vi "VPA QC Pressure Test.vi"(7 "DAQ Q":T1, 9 "DAQ Ref Cluster":T2, 10 "State Cluster":T3) -> (2 "State Cluster Out":T3)   [LabVIEW 2013]
uses:
  Controls/VPA QC State Data Cluster.ctl
  Controls/VPA QC General Cluster.ctl
  Controls/VPA QC State Enum.ctl
  Controls/VPA QC Bool Cluster.ctl
  Controls/VPA QC DAQ Ref Cluster.ctl
  Controls/VPA QC DAQ Q.ctl
  Controls/VPA QC DAQ Cmd Enum.ctl
panel:
  in  "Cancel":bool
  in  "Save":bool
  in  "Stop Logging":bool
  in  "Log":bool
  out "Pressure Test":dbl[][](graph)
  # "Pressure Verification Test"
  # "1. In pressure control mode, ramp to 95% max pressure."
  # "2. Start logging"
  # "3. Crack the external valve enough to allow the cylinders to transition twice."
  # "Assembly Checklist"
  # "Assembly Checklist"
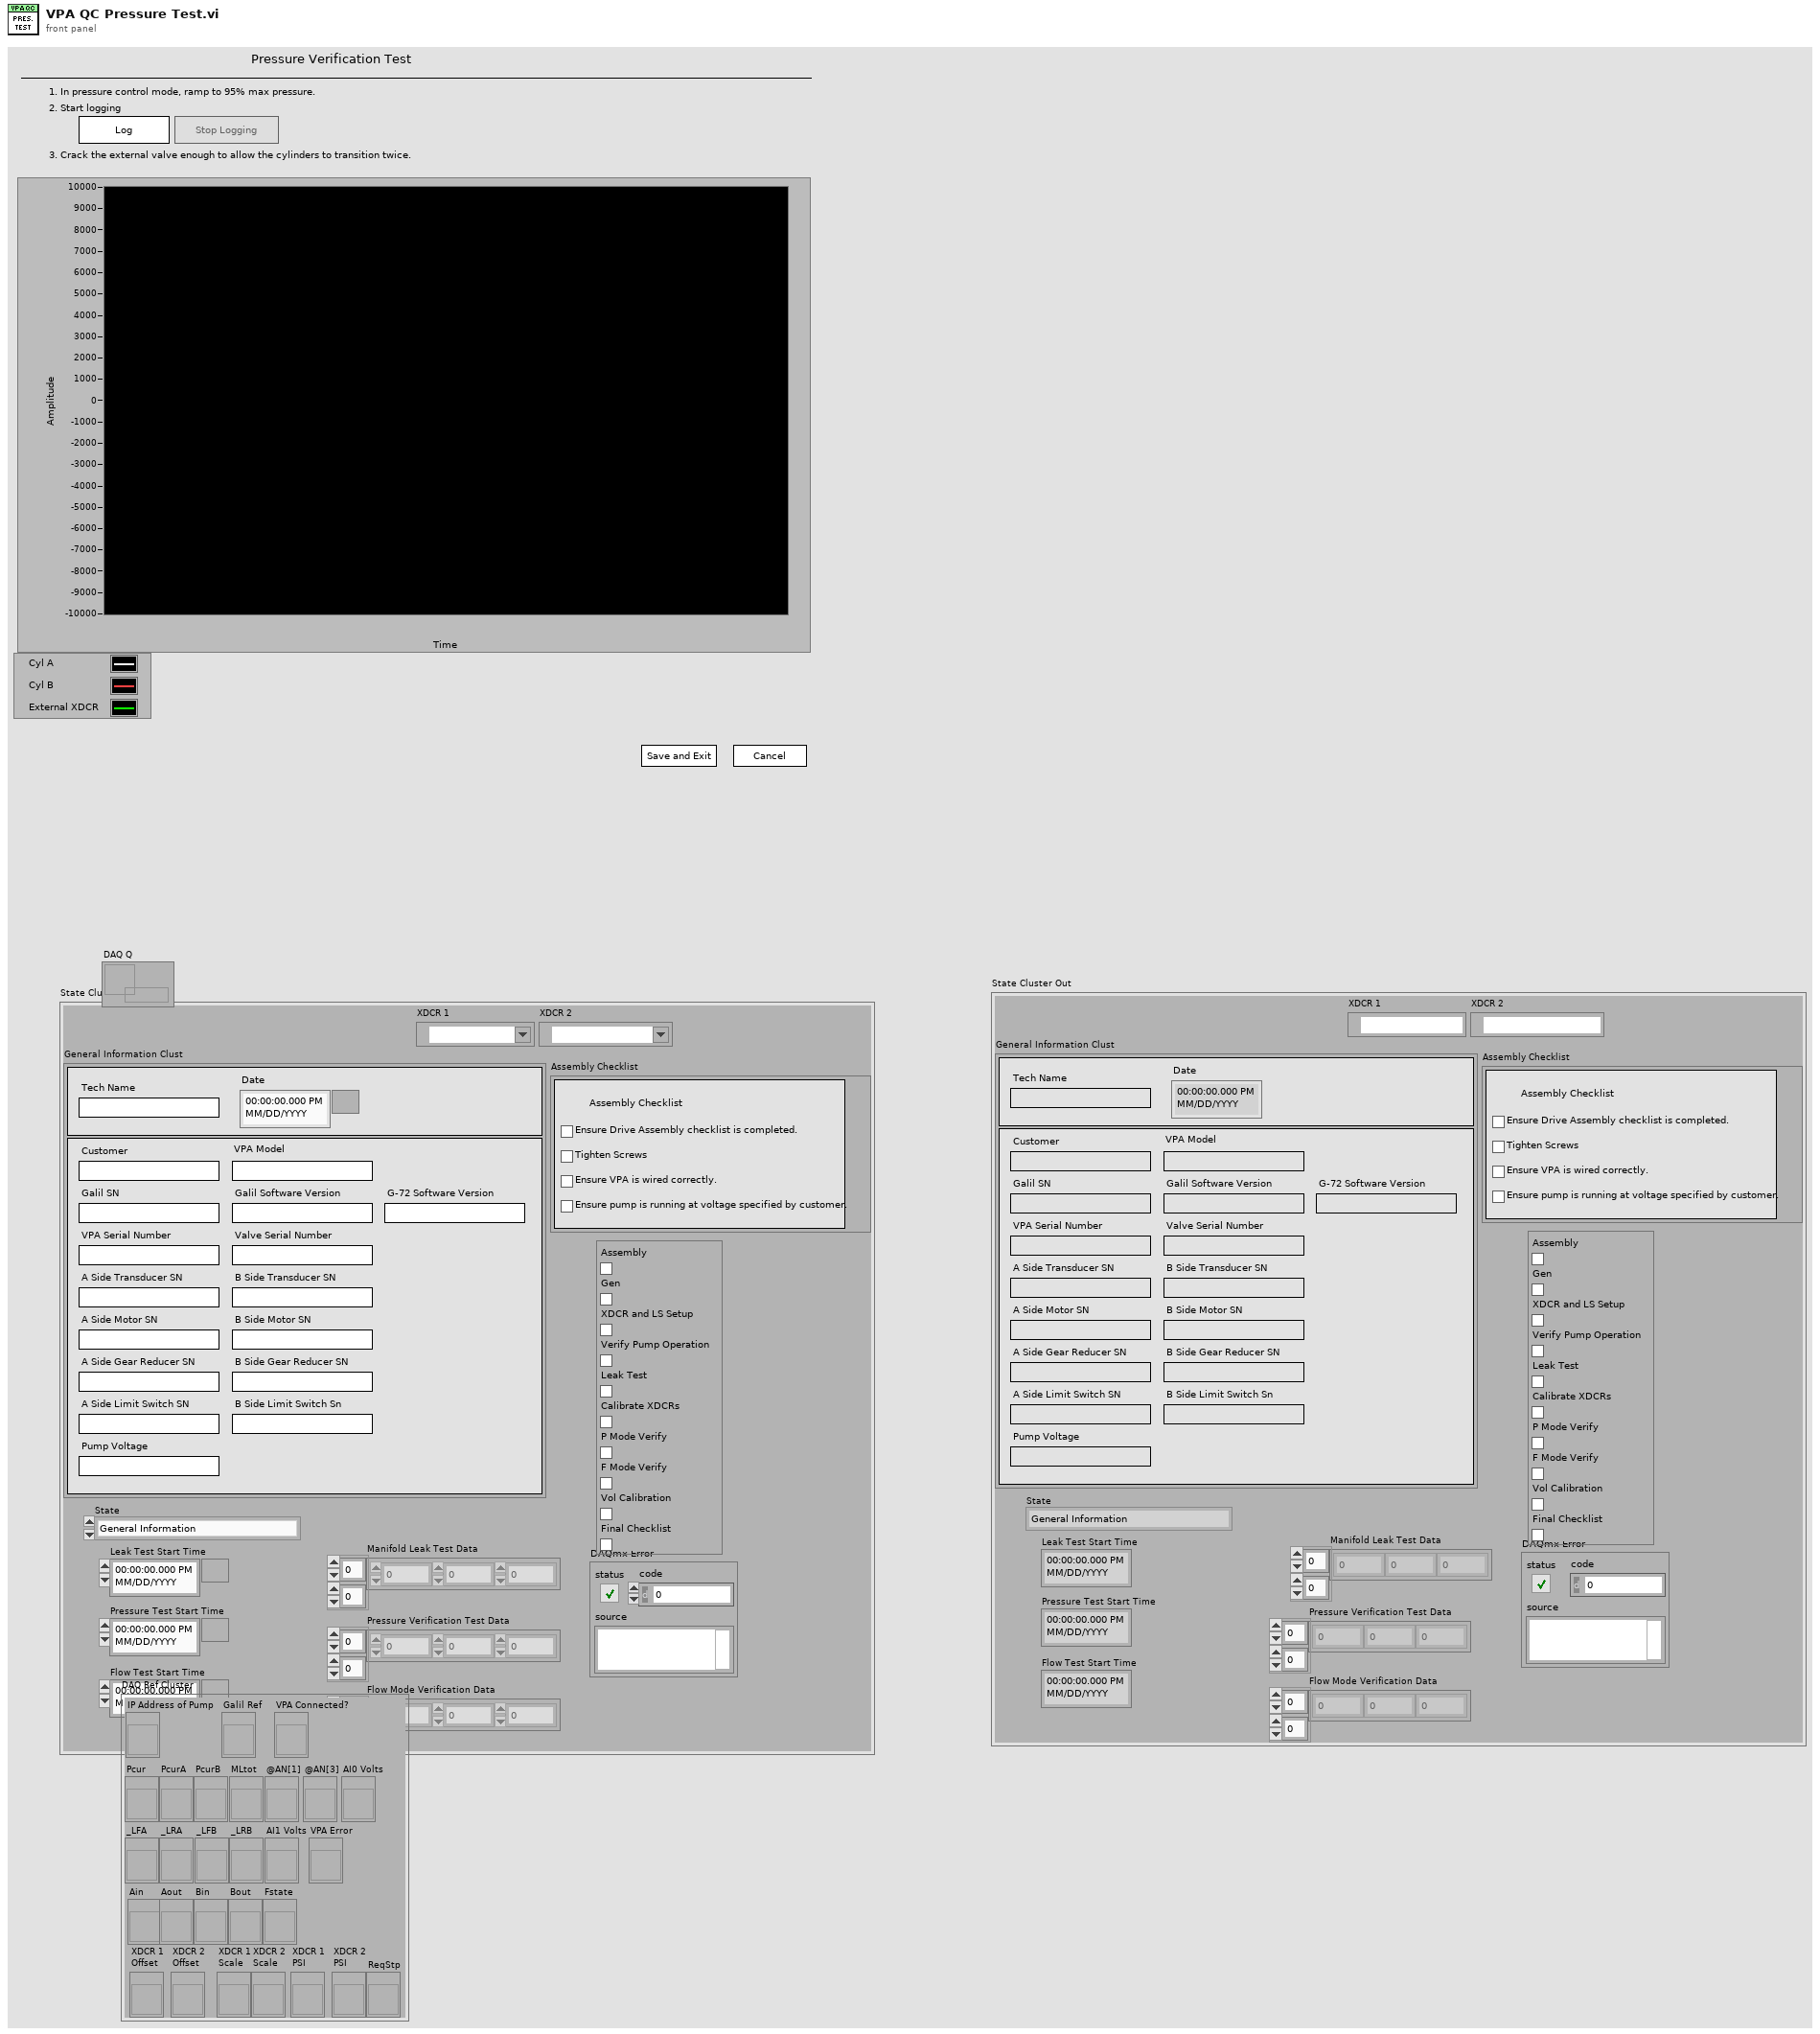
[diagram p1: front panel]
types:
  T1 = typedef "VPA QC DAQ Q.ctl" = refnum<queue>
  T2 = typedef "VPA QC DAQ Ref Cluster.ctl" = cluster{"IP Address of Pump":refnum<vi>, "Galil Ref":refnum<vi>, "VPA Connected?":refnum<vi>, "Pcur":refnum<vi>, "PcurA":refnum<vi>, "PcurB":refnum<vi>, "MLtot":refnum<vi>, "_LFA":refnum<vi>, "_LRA":refnum<vi>, "_LFB":refnum<vi>, "_LRB":refnum<vi>, "@AN[1]":refnum<vi>, "@AN[3]":refnum<vi>, "AI0 Volts":refnum<vi>, "AI1 Volts":refnum<vi>, "VPA Error":refnum<vi>, "Ain":refnum<vi>, "Aout":refnum<vi>, "Bin":refnum<vi>, "Bout":refnum<vi>, "Fstate":refnum<vi>, "XDCR 1\nOffset":refnum<vi>, "XDCR 2 \nOffset":refnum<vi>, "XDCR 1\nScale":refnum<vi>, "XDCR 2\nScale":refnum<vi>, "XDCR 1\nPSI":refnum<vi>, "XDCR 2\nPSI":refnum<vi>, "ReqStp":refnum<vi>}
  T3 = typedef "VPA QC State Data Cluster.ctl" = cluster{"XDCR 1":tag, "XDCR 2":tag, "General Information Clust":T4, "Assembly Checklist":cluster{"Ensure Drive Assembly checklist is completed.":bool, "Tighten Screws":bool, "Ensure VPA is wired correctly.":bool, "Ensure pump is running at voltage specified by customer.":bool}, "State":T5, "Manifold Leak Test Data":dbl[][], "Pressure Verification Test Data":dbl[][], "Flow Mode Verification Data":dbl[][], "DAQmx Error":errorcluster, "Bool Cluster":T6, "Leak Test Start Time":timestamp, "Pressure Test Start Time":timestamp, "Flow Test Start Time":timestamp}
  T4 = typedef "VPA QC General Cluster.ctl" = cluster{"Tech Name":string, "Customer":string, "VPA Model":string, "Galil SN":string, "Galil Software Version":string, "G-72 Software Version":string, "VPA Serial Number":string, "Valve Serial Number":string, "A Side Transducer SN":string, "B Side Transducer SN":string, "A Side Motor SN":string, "B Side Motor SN":string, "A Side Gear Reducer SN":string, "B Side Gear Reducer SN":string, "A Side Limit Switch SN":string, "B Side Limit Switch Sn":string, "Pump Voltage":string, "Date":timestamp}
  T5 = typedef "VPA QC State Enum.ctl" = enum16{"General Information", "XDCR and LS Check", "Check Pump Function", "Manifold/Cylinder Leak Test", "Exit"}
  T6 = typedef "VPA QC Bool Cluster.ctl" = cluster{"Assembly":bool, "Gen":bool, "XDCR and LS Setup":bool, "Verify Pump Operation":bool, "Leak Test":bool, "Calibrate XDCRs":bool, "P Mode Verify":bool, "F Mode Verify":bool, "Vol Calibration":bool, "Final Checklist":bool}
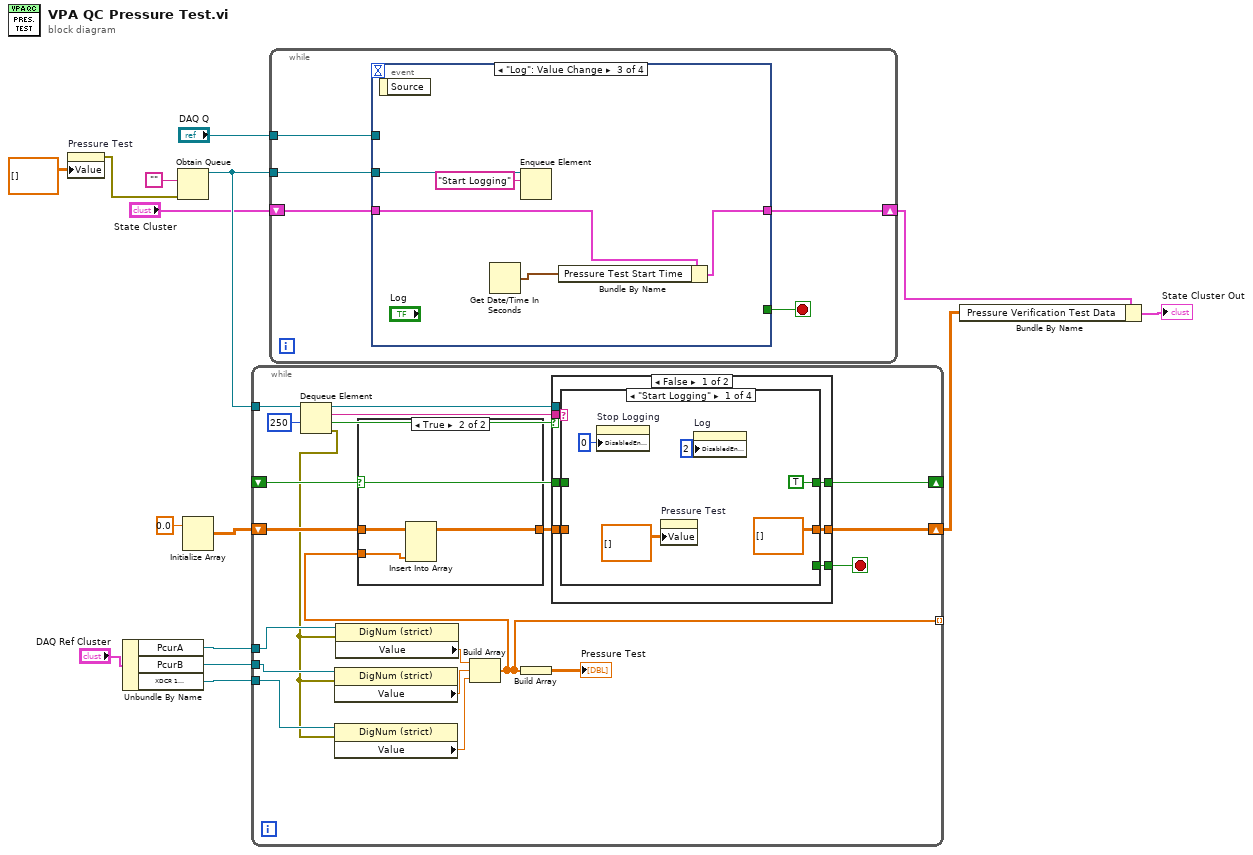
[diagram p0: block diagram]
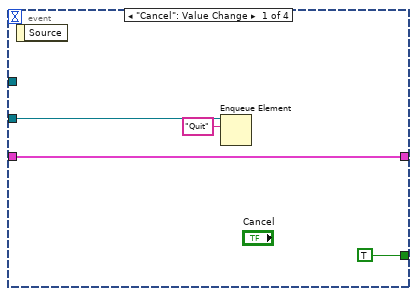
[diagram p2: hidden frame]
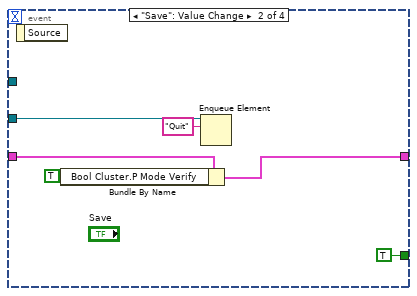
[diagram p3: hidden frame]
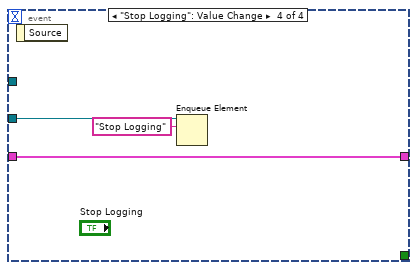
[diagram p4: hidden frame]
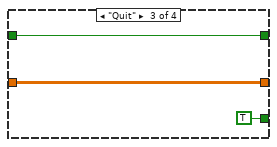
[diagram p7: hidden frame]
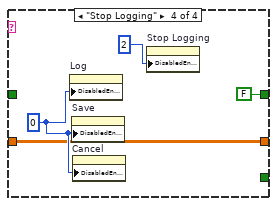
[diagram p8: hidden frame]
diagram:
  n1 = property on="Pressure Test" class="WFChart (strict)"("Value"=dbl[][] [] ("Pressure Test")) -> (error out=w1:errorcluster)  [unwired: 2 in, 1 out]
  n2 = Unbundle By Name("DAQ Ref Cluster") -> ("PcurA"=w14:refnum<vi>, "PcurB"=w13:refnum<vi>, "XDCR 1\nPSI"=w4:refnum<vi>)
  n3 = Obtain Queue(element data type="", error in (no error)=w1) -> (queue out=w11:refnum<queue>)  [unwired: 3 in, 2 out]
  n4 = Initialize Array(0.0 ("element")) -> (w10:dbl[][])  [unwired: 2 in]
  n5 = while {
    tunnel: w14 -> [w34]
    tunnel: w13 -> [w35]
    tunnel: w11 -> [w31]
    shift-right: [w26] -> _
    shift-left: _ -> [w24]
    shift-right: [w22] -> w3
    shift-left: w10 -> [w25]
    tunnel: w4 -> [w20]
    tunnel: [w16] -> _ mode=indexing
    stop <- w27 stop-if-true
    n6 = Dequeue Element(queue=w31, timeout in ms (-1)=250) -> (queue out=w21:refnum<queue>, element=w29:string, timed out?=w28:bool, error out=w19:errorcluster)  [unwired: 1 in]
    n7 = property class="DigNum (strict)"(reference=w35, error in=w19) -> ("Value"=w32:dbl)  [unwired: 2 out]
    n8 = property class="DigNum (strict)"(reference=w20, error in=w19) -> ("Value"=w18:dbl)  [unwired: 2 out]
    n9 = property class="DigNum (strict)"(reference=w34, error in=w19) -> ("Value"=w33:dbl)  [unwired: 2 out]
    n10 = Build Array(w33, w32, w18) -> (w16:dbl[])
    n11 = case shown="True" w24 {
      tunnel: w16 -> [_ w38]
      tunnel: w25 -> [w36 w39]
      tunnel: [w36 w37] -> w23
      frame False {
      }
      frame True {
        n12 = Insert Into Array(array=w39, new element=w38) -> (w37:dbl[][])  [unwired: 2 in]
      }
    }
    n13 = Build Array(w16) -> (→"Pressure Test":dbl[][])
    n14 = case shown="False" w28 {
      tunnel: w29 -> [w45 _]
      tunnel: [w44 _] -> w27
      tunnel: [w43 w61] -> w26
      tunnel: w24 -> [w42 w61]
      tunnel: w23 -> [w41 w60]
      tunnel: [w40 w60] -> w22
      tunnel: w21 -> [_ _]
      frame False {
        n15 = case shown="\"Start Logging\"" w45 {
          tunnel: [_ _ TRUE _] -> w44
          tunnel: [TRUE w52 w54 FALSE] -> w43
          tunnel: w42 -> [_ w52 w54 _]
          tunnel: w41 -> [_ w51 w53 w56]
          tunnel: [dbl[][] [] w51 w53 w56] -> w40
          frame "Start Logging" {
            n16 = property on="Stop Logging" class="Bool"("DisabledEnum"=u8 0) -> ()  [unwired: 2 in, 2 out]
            n17 = property on="Pressure Test" class="WFChart (strict)"("Value"=dbl[][] [] ("Pressure Test")) -> ()  [unwired: 2 in, 2 out]
            n18 = property on="Log" class="Bool"("DisabledEnum"=u8 2) -> ()  [unwired: 2 in, 2 out]
          }
          frame Default {
          }
          frame "Quit" {
          }
          frame "Stop Logging" {
            w58 = u8 0
            n19 = property on="Log" class="Bool"("DisabledEnum"=w58) -> ()  [unwired: 2 in, 2 out]
            n20 = property on="Save" class="Bool"("DisabledEnum"=w58) -> ()  [unwired: 2 in, 2 out]
            n21 = property on="Cancel" class="Bool"("DisabledEnum"=w58) -> ()  [unwired: 2 in, 2 out]
            n22 = property on="Stop Logging" class="Bool"("DisabledEnum"=u8 2) -> ()  [unwired: 2 in, 2 out]
          }
        }
      }
      frame True {
      }
    }
  }
  n23 = while {
    tunnel: w11 -> [w65]
    shift-right: [w63] -> w6
    shift-left: "State Cluster" -> [w64]
    tunnel: "DAQ Q" -> [w62]
    stop <- w66 stop-if-true
    n24 = event shown="[2] \"Log\": Value Change" {
      selector: _ -> [_ _ _ _]
      dyn-events: _ -> [_ _ _ _]
      timeout: _ -> [_ _ _ _]
      tunnel: [TRUE TRUE _ _] -> w66
      tunnel: w65 -> [w69 w72 w81 w84]
      tunnel: w64 -> [w67 w75 w78 w82]
      tunnel: [w67 w73 w77 w82] -> w63
      tunnel: w62 -> [_ _ _ _]
      event "Cancel": Value Change {
        n25 = event-data() -> ()  [unwired: 1 in, 1 out]
        n26 = Enqueue Element(queue=w69, element="Quit") -> ()  [unwired: 2 in, 3 out]
      }
      event "Save": Value Change {
        n27 = event-data() -> ()  [unwired: 1 in, 1 out]
        n28 = Bundle By Name(cluster=w75, "Bool Cluster.P Mode Verify"=TRUE ("Bool Cluster.Leak Test")) -> (w73:T3)
        n29 = Enqueue Element(queue=w72, element="Quit") -> ()  [unwired: 2 in, 3 out]
      }
      event "Log": Value Change {
        n30 = event-data() -> ()  [unwired: 1 in, 1 out]
        n31 = Get Date/Time In Seconds() -> (seconds since 1Jan1904=w79:timestamp)
        n32 = Enqueue Element(queue=w81, element="Start Logging") -> ()  [unwired: 2 in, 3 out]
        n33 = Bundle By Name(cluster=w78, "Pressure Test Start Time"=w79) -> (w77:T3)
      }
      event "Stop Logging": Value Change {
        n34 = event-data() -> ()  [unwired: 1 in, 1 out]
        n35 = Enqueue Element(queue=w84, element="Stop Logging") -> ()  [unwired: 2 in, 3 out]
      }
    }
  }
  n36 = Bundle By Name(cluster=w6, "Pressure Verification Test Data"=w3) -> (→"State Cluster Out":T3)
